vi "Get band variation.vi"(9 "# taps / position":i32=1, 10 "Bands 2":u16(ring)=2 items=["No Bands", "JC violin 200-7000 Flat (200-7000)", "JC violin (200-780-1740-2930-7000)", "JC violin (200-780-7000)", "MJ_Test (200-428-453-780-1740-2930-7000)"], 11 "Files":path[](array[path])=[path "/Users/crogers/Dropbox (Rogers)/Violin Stuff/PC ViolnData/SoundCard2/SoundCard2 ModalShop7/Raw/SoundCard2 ModalShop7 H_001_001.wfm", path "/Users/crogers/Dropbox (Rogers)/Violin Stuff/PC ViolnData/SoundCard2/SoundCard2 ModalShop7/Raw/SoundCard2 ModalShop7 H_001_002.wfm", path "/Users/crogers/Dropbox (Rogers)/Violin Stuff/PC ViolnData/SoundCard2/SoundCard2 ModalShop7/Raw/SoundCard2 ModalShop7 H_001_003.wfm", path "/Users/crogers/Dropbox (Rogers)/Violin Stuff/PC ViolnData/SoundCard2/SoundCard2 ModalShop7/Raw/SoundCard2 ModalShop7 H_001_004.wfm", path "/Users/crogers/Dropbox (Rogers)/Violin Stuff/PC ViolnData/SoundCard2/SoundCard2 ModalShop7/Raw/SoundCard2 ModalShop7 H_001_005.wfm", path "/Users/crogers/Dropbox (Rogers)/Violin Stuff/PC ViolnData/SoundCard2/SoundCard2 ModalShop7/Raw/SoundCard2 ModalShop7 H_001_006.wfm", path "/Users/crogers/Dropbox (Rogers)/Violin Stuff/PC ViolnData/SoundCard2/SoundCard2 ModalShop7/Raw/SoundCard2 ModalShop7 H_001_007.wfm", path "/Users/crogers/Dropbox (Rogers)/Violin Stuff/PC ViolnData/SoundCard2/SoundCard2 ModalShop7/Raw/SoundCard2 ModalShop7 H_001_008.wfm", path "/Users/crogers/Dropbox (Rogers)/Violin Stuff/PC ViolnData/SoundCard2/SoundCard2 ModalShop7/Raw/SoundCard2 ModalShop7 H_001_009.wfm", path "/Users/crogers/Dropbox (Rogers)/Violin Stuff/PC ViolnData/SoundCard2/SoundCard2 ModalShop7/Raw/SoundCard2 ModalShop7 H_001_010.wfm", path "/Users/crogers/Dropbox (Rogers)/Violin Stuff/PC ViolnData/SoundCard2/SoundCard2 ModalShop7/Raw/SoundCard2 ModalShop7 H_002_001.wfm", path "/Users/crogers/Dropbox (Rogers)/Violin Stuff/PC ViolnData/SoundCard2/SoundCard2 ModalShop7/Raw/SoundCard2 ModalShop7 H_002_002.wfm", path "/Users/crogers/Dropbox (Rogers)/Violin Stuff/PC ViolnData/SoundCard2/SoundCard2 ModalShop7/Raw/SoundCard2 ModalShop7 H_002_003.wfm", path "/Users/crogers/Dropbox (Rogers)/Violin Stuff/PC ViolnData/SoundCard2/SoundCard2 ModalShop7/Raw/SoundCard2 ModalShop7 H_002_004.wfm", path "/Users/crogers/Dropbox (Rogers)/Violin Stuff/PC ViolnData/SoundCard2/SoundCard2 ModalShop7/Raw/SoundCard2 ModalShop7 H_002_005.wfm", path "/Users/crogers/Dropbox (Rogers)/Violin Stuff/PC ViolnData/SoundCard2/SoundCard2 ModalShop7/Raw/SoundCard2 ModalShop7 H_002_006.wfm", path "/Users/crogers/Dropbox (Rogers)/Violin Stuff/PC ViolnData/SoundCard2/SoundCard2 ModalShop7/Raw/SoundCard2 ModalShop7 H_002_007.wfm", path "/Users/crogers/Dropbox (Rogers)/Violin Stuff/PC ViolnData/SoundCard2/SoundCard2 ModalShop7/Raw/SoundCard2 ModalShop7 H_002_008.wfm", path "/Users/crogers/Dropbox (Rogers)/Violin Stuff/PC ViolnData/SoundCard2/SoundCard2 ModalShop7/Raw/SoundCard2 ModalShop7 H_002_009.wfm", path "/Users/crogers/Dropbox (Rogers)/Violin Stuff/PC ViolnData/SoundCard2/SoundCard2 ModalShop7/Raw/SoundCard2 ModalShop7 H_002_010.wfm", path "/Users/crogers/Dropbox (Rogers)/Violin Stuff/PC ViolnData/SoundCard2/SoundCard2 ModalShop7/Raw/SoundCard2 ModalShop7 H_003_001.wfm", path "/Users/crogers/Dropbox (Rogers)/Violin Stuff/PC ViolnData/SoundCard2/SoundCard2 ModalShop7/Raw/SoundCard2 ModalShop7 H_003_002.wfm", path "/Users/crogers/Dropbox (Rogers)/Violin Stuff/PC ViolnData/SoundCard2/SoundCard2 ModalShop7/Raw/SoundCard2 ModalShop7 H_003_003.wfm", path "/Users/crogers/Dropbox (Rogers)/Violin Stuff/PC ViolnData/SoundCard2/SoundCard2 ModalShop7/Raw/SoundCard2 ModalShop7 H_003_004.wfm", path "/Users/crogers/Dropbox (Rogers)/Violin Stuff/PC ViolnData/SoundCard2/SoundCard2 ModalShop7/Raw/SoundCard2 ModalShop7 H_003_005.wfm", path "/Users/crogers/Dropbox (Rogers)/Violin Stuff/PC ViolnData/SoundCard2/SoundCard2 ModalShop7/Raw/SoundCard2 ModalShop7 H_003_006.wfm", path "/Users/crogers/Dropbox (Rogers)/Violin Stuff/PC ViolnData/SoundCard2/SoundCard2 ModalShop7/Raw/SoundCard2 ModalShop7 H_003_007.wfm", path "/Users/crogers/Dropbox (Rogers)/Violin Stuff/PC ViolnData/SoundCard2/SoundCard2 ModalShop7/Raw/SoundCard2 ModalShop7 H_003_008.wfm", path "/Users/crogers/Dropbox (Rogers)/Violin Stuff/PC ViolnData/SoundCard2/SoundCard2 ModalShop7/Raw/SoundCard2 ModalShop7 H_003_009.wfm", path "/Users/crogers/Dropbox (Rogers)/Violin Stuff/PC ViolnData/SoundCard2/SoundCard2 ModalShop7/Raw/SoundCard2 ModalShop7 H_003_010.wfm", path "/Users/crogers/Dropbox (Rogers)/Violin Stuff/PC ViolnData/SoundCard2/SoundCard2 ModalShop7/Raw/SoundCard2 ModalShop7 H_004_001.wfm", path "/Users/crogers/Dropbox (Rogers)/Violin Stuff/PC ViolnData/SoundCard2/SoundCard2 ModalShop7/Raw/SoundCard2 ModalShop7 H_004_002.wfm", path "/Users/crogers/Dropbox (Rogers)/Violin Stuff/PC ViolnData/SoundCard2/SoundCard2 ModalShop7/Raw/SoundCard2 ModalShop7 H_004_003.wfm", path "/Users/crogers/Dropbox (Rogers)/Violin Stuff/PC ViolnData/SoundCard2/SoundCard2 ModalShop7/Raw/SoundCard2 ModalShop7 H_004_004.wfm", path "/Users/crogers/Dropbox (Rogers)/Violin Stuff/PC ViolnData/SoundCard2/SoundCard2 ModalShop7/Raw/SoundCard2 ModalShop7 H_004_005.wfm", path "/Users/crogers/Dropbox (Rogers)/Violin Stuff/PC ViolnData/SoundCard2/SoundCard2 ModalShop7/Raw/SoundCard2 ModalShop7 H_004_006.wfm", path "/Users/crogers/Dropbox (Rogers)/Violin Stuff/PC ViolnData/SoundCard2/SoundCard2 ModalShop7/Raw/SoundCard2 ModalShop7 H_004_007.wfm", path "/Users/crogers/Dropbox (Rogers)/Violin Stuff/PC ViolnData/SoundCard2/SoundCard2 ModalShop7/Raw/SoundCard2 ModalShop7 H_004_008.wfm", path "/Users/crogers/Dropbox (Rogers)/Violin Stuff/PC ViolnData/SoundCard2/SoundCard2 ModalShop7/Raw/SoundCard2 ModalShop7 H_004_009.wfm", path "/Users/crogers/Dropbox (Rogers)/Violin Stuff/PC ViolnData/SoundCard2/SoundCard2 ModalShop7/Raw/SoundCard2 ModalShop7 H_004_010.wfm", path "/Users/crogers/Dropbox (Rogers)/Violin Stuff/PC ViolnData/SoundCard2/SoundCard2 ModalShop7/Raw/SoundCard2 ModalShop7 H_005_001.wfm", path "/Users/crogers/Dropbox (Rogers)/Violin Stuff/PC ViolnData/SoundCard2/SoundCard2 ModalShop7/Raw/SoundCard2 ModalShop7 H_005_002.wfm", path "/Users/crogers/Dropbox (Rogers)/Violin Stuff/PC ViolnData/SoundCard2/SoundCard2 ModalShop7/Raw/SoundCard2 ModalShop7 H_005_003.wfm", path "/Users/crogers/Dropbox (Rogers)/Violin Stuff/PC ViolnData/SoundCard2/SoundCard2 ModalShop7/Raw/SoundCard2 ModalShop7 H_005_004.wfm", path "/Users/crogers/Dropbox (Rogers)/Violin Stuff/PC ViolnData/SoundCard2/SoundCard2 ModalShop7/Raw/SoundCard2 ModalShop7 H_005_005.wfm", path "/Users/crogers/Dropbox (Rogers)/Violin Stuff/PC ViolnData/SoundCard2/SoundCard2 ModalShop7/Raw/SoundCard2 ModalShop7 H_005_006.wfm", path "/Users/crogers/Dropbox (Rogers)/Violin Stuff/PC ViolnData/SoundCard2/SoundCard2 ModalShop7/Raw/SoundCard2 ModalShop7 H_005_007.wfm", path "/Users/crogers/Dropbox (Rogers)/Violin Stuff/PC ViolnData/SoundCard2/SoundCard2 ModalShop7/Raw/SoundCard2 ModalShop7 H_005_008.wfm", path "/Users/crogers/Dropbox (Rogers)/Violin Stuff/PC ViolnData/SoundCard2/SoundCard2 ModalShop7/Raw/SoundCard2 ModalShop7 H_005_009.wfm", path "/Users/crogers/Dropbox (Rogers)/Violin Stuff/PC ViolnData/SoundCard2/SoundCard2 ModalShop7/Raw/SoundCard2 ModalShop7 H_005_010.wfm", path "/Users/crogers/Dropbox (Rogers)/Violin Stuff/PC ViolnData/SoundCard2/SoundCard2 ModalShop8/Raw/SoundCard2 ModalShop8 H_001_001.wfm", path "/Users/crogers/Dropbox (Rogers)/Violin Stuff/PC ViolnData/SoundCard2/SoundCard2 ModalShop8/Raw/SoundCard2 ModalShop8 H_001_002.wfm", path "/Users/crogers/Dropbox (Rogers)/Violin Stuff/PC ViolnData/SoundCard2/SoundCard2 ModalShop8/Raw/SoundCard2 ModalShop8 H_001_003.wfm", path "/Users/crogers/Dropbox (Rogers)/Violin Stuff/PC ViolnData/SoundCard2/SoundCard2 ModalShop8/Raw/SoundCard2 ModalShop8 H_001_004.wfm", path "/Users/crogers/Dropbox (Rogers)/Violin Stuff/PC ViolnData/SoundCard2/SoundCard2 ModalShop8/Raw/SoundCard2 ModalShop8 H_001_005.wfm", path "/Users/crogers/Dropbox (Rogers)/Violin Stuff/PC ViolnData/SoundCard2/SoundCard2 ModalShop8/Raw/SoundCard2 ModalShop8 H_001_006.wfm", path "/Users/crogers/Dropbox (Rogers)/Violin Stuff/PC ViolnData/SoundCard2/SoundCard2 ModalShop8/Raw/SoundCard2 ModalShop8 H_001_007.wfm", path "/Users/crogers/Dropbox (Rogers)/Violin Stuff/PC ViolnData/SoundCard2/SoundCard2 ModalShop8/Raw/SoundCard2 ModalShop8 H_001_008.wfm", path "/Users/crogers/Dropbox (Rogers)/Violin Stuff/PC ViolnData/SoundCard2/SoundCard2 ModalShop8/Raw/SoundCard2 ModalShop8 H_001_009.wfm", path "/Users/crogers/Dropbox (Rogers)/Violin Stuff/PC ViolnData/SoundCard2/SoundCard2 ModalShop8/Raw/SoundCard2 ModalShop8 H_001_010.wfm", path "/Users/crogers/Dropbox (Rogers)/Violin Stuff/PC ViolnData/SoundCard2/SoundCard2 ModalShop8/Raw/SoundCard2 ModalShop8 H_002_001.wfm", path "/Users/crogers/Dropbox (Rogers)/Violin Stuff/PC ViolnData/SoundCard2/SoundCard2 ModalShop8/Raw/SoundCard2 ModalShop8 H_002_002.wfm", path "/Users/crogers/Dropbox (Rogers)/Violin Stuff/PC ViolnData/SoundCard2/SoundCard2 ModalShop8/Raw/SoundCard2 ModalShop8 H_002_003.wfm", path "/Users/crogers/Dropbox (Rogers)/Violin Stuff/PC ViolnData/SoundCard2/SoundCard2 ModalShop8/Raw/SoundCard2 ModalShop8 H_002_004.wfm", path "/Users/crogers/Dropbox (Rogers)/Violin Stuff/PC ViolnData/SoundCard2/SoundCard2 ModalShop8/Raw/SoundCard2 ModalShop8 H_002_005.wfm", path "/Users/crogers/Dropbox (Rogers)/Violin Stuff/PC ViolnData/SoundCard2/SoundCard2 ModalShop8/Raw/SoundCard2 ModalShop8 H_002_006.wfm", path "/Users/crogers/Dropbox (Rogers)/Violin Stuff/PC ViolnData/SoundCard2/SoundCard2 ModalShop8/Raw/SoundCard2 ModalShop8 H_002_007.wfm", path "/Users/crogers/Dropbox (Rogers)/Violin Stuff/PC ViolnData/SoundCard2/SoundCard2 ModalShop8/Raw/SoundCard2 ModalShop8 H_002_008.wfm", path "/Users/crogers/Dropbox (Rogers)/Violin Stuff/PC ViolnData/SoundCard2/SoundCard2 ModalShop8/Raw/SoundCard2 ModalShop8 H_002_009.wfm", path "/Users/crogers/Dropbox (Rogers)/Violin Stuff/PC ViolnData/SoundCard2/SoundCard2 ModalShop8/Raw/SoundCard2 ModalShop8 H_002_010.wfm", path "/Users/crogers/Dropbox (Rogers)/Violin Stuff/PC ViolnData/SoundCard2/SoundCard2 ModalShop8/Raw/SoundCard2 ModalShop8 H_003_001.wfm", path "/Users/crogers/Dropbox (Rogers)/Violin Stuff/PC ViolnData/SoundCard2/SoundCard2 ModalShop8/Raw/SoundCard2 ModalShop8 H_003_002.wfm", path "/Users/crogers/Dropbox (Rogers)/Violin Stuff/PC ViolnData/SoundCard2/SoundCard2 ModalShop8/Raw/SoundCard2 ModalShop8 H_003_003.wfm", path "/Users/crogers/Dropbox (Rogers)/Violin Stuff/PC ViolnData/SoundCard2/SoundCard2 ModalShop8/Raw/SoundCard2 ModalShop8 H_003_004.wfm", path "/Users/crogers/Dropbox (Rogers)/Violin Stuff/PC ViolnData/SoundCard2/SoundCard2 ModalShop8/Raw/SoundCard2 ModalShop8 H_003_005.wfm", path "/Users/crogers/Dropbox (Rogers)/Violin Stuff/PC ViolnData/SoundCard2/SoundCard2 ModalShop8/Raw/SoundCard2 ModalShop8 H_003_006.wfm", path "/Users/crogers/Dropbox (Rogers)/Violin Stuff/PC ViolnData/SoundCard2/SoundCard2 ModalShop8/Raw/SoundCard2 ModalShop8 H_003_007.wfm", path "/Users/crogers/Dropbox (Rogers)/Violin Stuff/PC ViolnData/SoundCard2/SoundCard2 ModalShop8/Raw/SoundCard2 ModalShop8 H_003_008.wfm", path "/Users/crogers/Dropbox (Rogers)/Violin Stuff/PC ViolnData/SoundCard2/SoundCard2 ModalShop8/Raw/SoundCard2 ModalShop8 H_003_009.wfm", path "/Users/crogers/Dropbox (Rogers)/Violin Stuff/PC ViolnData/SoundCard2/SoundCard2 ModalShop8/Raw/SoundCard2 ModalShop8 H_003_010.wfm", path "/Users/crogers/Dropbox (Rogers)/Violin Stuff/PC ViolnData/SoundCard2/SoundCard2 ModalShop8/Raw/SoundCard2 ModalShop8 H_004_001.wfm", path "/Users/crogers/Dropbox (Rogers)/Violin Stuff/PC ViolnData/SoundCard2/SoundCard2 ModalShop8/Raw/SoundCard2 ModalShop8 H_004_002.wfm", path "/Users/crogers/Dropbox (Rogers)/Violin Stuff/PC ViolnData/SoundCard2/SoundCard2 ModalShop8/Raw/SoundCard2 ModalShop8 H_004_003.wfm", path "/Users/crogers/Dropbox (Rogers)/Violin Stuff/PC ViolnData/SoundCard2/SoundCard2 ModalShop8/Raw/SoundCard2 ModalShop8 H_004_004.wfm", path "/Users/crogers/Dropbox (Rogers)/Violin Stuff/PC ViolnData/SoundCard2/SoundCard2 ModalShop8/Raw/SoundCard2 ModalShop8 H_004_005.wfm", path "/Users/crogers/Dropbox (Rogers)/Violin Stuff/PC ViolnData/SoundCard2/SoundCard2 ModalShop8/Raw/SoundCard2 ModalShop8 H_004_006.wfm", path "/Users/crogers/Dropbox (Rogers)/Violin Stuff/PC ViolnData/SoundCard2/SoundCard2 ModalShop8/Raw/SoundCard2 ModalShop8 H_004_007.wfm", path "/Users/crogers/Dropbox (Rogers)/Violin Stuff/PC ViolnData/SoundCard2/SoundCard2 ModalShop8/Raw/SoundCard2 ModalShop8 H_004_008.wfm", path "/Users/crogers/Dropbox (Rogers)/Violin Stuff/PC ViolnData/SoundCard2/SoundCard2 ModalShop8/Raw/SoundCard2 ModalShop8 H_004_009.wfm", path "/Users/crogers/Dropbox (Rogers)/Violin Stuff/PC ViolnData/SoundCard2/SoundCard2 ModalShop8/Raw/SoundCard2 ModalShop8 H_004_010.wfm", path "/Users/crogers/Dropbox (Rogers)/Violin Stuff/PC ViolnData/SoundCard2/SoundCard2 ModalShop8/Raw/SoundCard2 ModalShop8 H_005_001.wfm", path "/Users/crogers/Dropbox (Rogers)/Violin Stuff/PC ViolnData/SoundCard2/SoundCard2 ModalShop8/Raw/SoundCard2 ModalShop8 H_005_002.wfm", path "/Users/crogers/Dropbox (Rogers)/Violin Stuff/PC ViolnData/SoundCard2/SoundCard2 ModalShop8/Raw/SoundCard2 ModalShop8 H_005_003.wfm", path "/Users/crogers/Dropbox (Rogers)/Violin Stuff/PC ViolnData/SoundCard2/SoundCard2 ModalShop8/Raw/SoundCard2 ModalShop8 H_005_004.wfm", path "/Users/crogers/Dropbox (Rogers)/Violin Stuff/PC ViolnData/SoundCard2/SoundCard2 ModalShop8/Raw/SoundCard2 ModalShop8 H_005_005.wfm", path "/Users/crogers/Dropbox (Rogers)/Violin Stuff/PC ViolnData/SoundCard2/SoundCard2 ModalShop8/Raw/SoundCard2 ModalShop8 H_005_006.wfm", path "/Users/crogers/Dropbox (Rogers)/Violin Stuff/PC ViolnData/SoundCard2/SoundCard2 ModalShop8/Raw/SoundCard2 ModalShop8 H_005_007.wfm", path "/Users/crogers/Dropbox (Rogers)/Violin Stuff/PC ViolnData/SoundCard2/SoundCard2 ModalShop8/Raw/SoundCard2 ModalShop8 H_005_008.wfm", path "/Users/crogers/Dropbox (Rogers)/Violin Stuff/PC ViolnData/SoundCard2/SoundCard2 ModalShop8/Raw/SoundCard2 ModalShop8 H_005_009.wfm", path "/Users/crogers/Dropbox (Rogers)/Violin Stuff/PC ViolnData/SoundCard2/SoundCard2 ModalShop8/Raw/SoundCard2 ModalShop8 H_005_010.wfm"]) -> (2 "sdev":dbl[](array[numeric]), 3 "mean":dbl[](array[numeric]))   [LabVIEW 2024]
uses:
  PreferencesControl.ctl
  <vilib>/Analysis/NI_AALBase.lvlib
panel:
  out "Histogram Graph":T1(graph)
  out "Bands 3":dbl[][](graph)
  out "Bands":cluster{dbl, "df":dbl, dbl[]}[](graph)
  out "Hammer Spectra":cluster{dbl, "df":dbl, "FFT {X}":dbl[]}[](graph)=[{0.0, "df"=1.0, "FFT {X}"=array[24001 elements]}]
  out "Microphone Spectra":cluster{"x0":dbl, "df":dbl, dbl[]}[](graph)=[{"x0"=0.0, "df"=1.0, array[24001 elements]}]
  out "Average FRF":cluster{dbl, "df":dbl, dbl[]}[](graph)=[{0.0, "df"=1.0, array[24001 elements]}, {0.0, "df"=1.0, array[24001 elements]}]
  out "Hammer":cluster{dbl, "dt":dbl, "Y":dbl[]}[](graph)=[{0.0, "dt"=2.0833333333333333e-05, "Y"=array[14400 elements]}]
  out "Microphone":cluster{dbl, "dt":dbl, "Y":dbl[]}[](graph)=[{0.0, "dt"=2.0833333333333333e-05, "Y"=array[14400 elements]}]
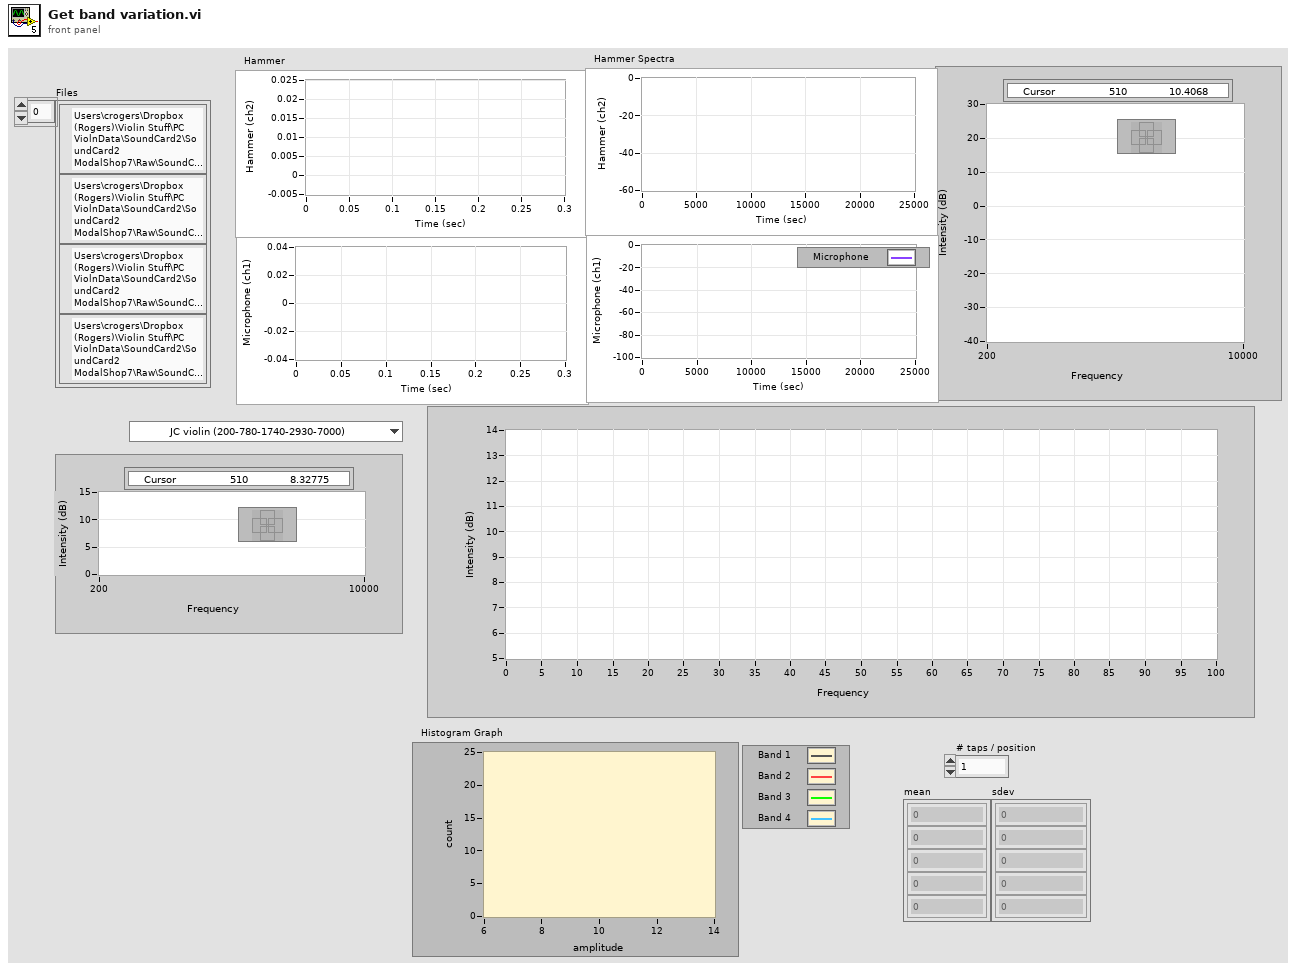
[diagram p1: front panel]
types:
  T1 = cluster{"X Values":dbl[], "Histogram: h(x)":i32[]}[]
  T2 = typedef "PreferencesControl.ctl" = cluster{"Name of test":string, "Date":timestamp, "Location":string, "Template":string, "Soundcard":string, "resolution":u16, "Sampling rate":u16, "Ch1 Gain ":dbl, "Ch2 Gain":dbl, "Sample time (s)":dbl, "Pre-trigger (s)":dbl, "Hammer Threshold":dbl, "Positions":i16, "Taps/Position":i16, "Set Names":string, "Freq resolution":dbl, "Hammer cutoff":dbl, "Mic cutoff":dbl, "Double bounce ":dbl, "Hammer Cal":dbl, "dB Offset":dbl, "Accel Cal":dbl, "Vibrometer Cal":dbl, "Mic Cal":dbl, "Output":u16, "Voltage Cal":dbl, "Vibrometer Port":refnum<visa-resource-name>, "Range":u16, "High Pass":u16, "Bandwidth":u16, "X Range":cluster{"Minimum":dbl, "Maximum":dbl, "Increment":dbl, "Minor Increment":dbl, "Start":dbl}[], "Y Range":cluster{"Minimum":dbl, "Maximum":dbl, "Increment":dbl, "Minor Increment":dbl, "Start":dbl}[], "dB Spread":dbl, "Trigger":u16, "Ch_1":u8, "Ch_2":u8, "flip?":bool, "60Hz":bool, "Time offset":dbl, "Piezo Cal":dbl, "Default Notes":string}
  T3 = cluster{"Name":string, "Color":u32, "Style":u8, "Point Style":u8, "Name Visible":bool, "Allow Drag":bool, "Cursor Mode":u32, "Plot":i32, "Index":i32, "Position":cluster{"X":dbl, "Y":dbl}, "X Scale":u32, "Y Scale":u32, "Watch Plots":i32[], "Watch All Plots":bool, "Plot Area":i32, "Label Offset":cluster{"X":dbl, "Y":dbl}}[]
  T4 = cluster{"Band ranges":dbl[][], "CoM":dbl[][], "Band Ave":dbl[][]}
  T5 = cluster{dbl, "df":dbl, "Power Spectrum (V^2 rms)":dbl[]}[]
  T6 = cluster{dbl, "df":dbl, "Power Spectrum (V^2 rms)":dbl[]}
  T7 = cluster{"X Values":dbl[], "Histogram: h(x)":i32[]}
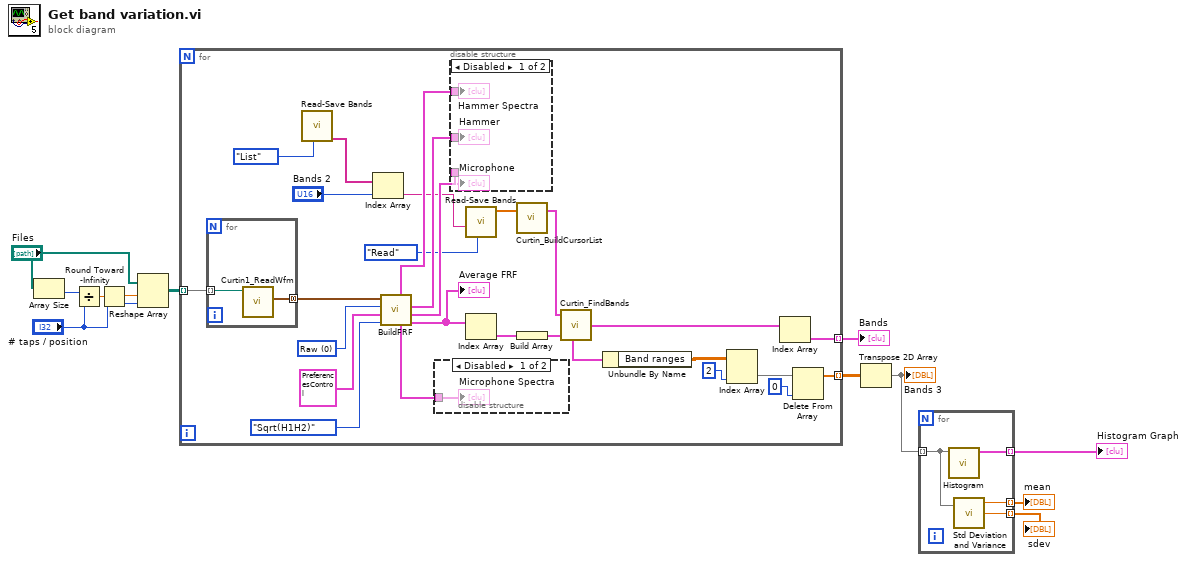
[diagram p0: block diagram]
diagram:
  n1 = Array Size(array="Files") -> (size(s)=w8:i32)
  n2 = Divide(x=w8, y="# taps / position") -> (x/y=w6:dbl)
  n3 = Round Toward -Infinity(1:w6) -> (0:w3:dbl)
  n4 = Reshape Array("Files", w3, "# taps / position") -> (w12:path[][])
  n5 = for {
    tunnel: w12 -> [w21] mode=indexing
    tunnel: [w19] -> w11 mode=indexing
    tunnel: [w14] -> w10 mode=indexing
    w38 = u16 0 items=["Raw", "Volts", "Units (Pa, N, mm/s etc)"] ("View")
    n6 = for {
      tunnel: [w45] -> w39 mode=concatenating
      tunnel: w21 -> [w44] mode=indexing
      n7 = call "Curtin1_ReadWfm.vi"("appended path"=w44) -> ("all waveforms in record"=w45:waveform(dbl)[])  [unwired: 9 in, 1 out]
    }
    n8 = call "Read-Save Bands.vi"("Task"=enum16{"Save", "Read", "List"}."List") -> ("file names"=w29:string[])  [unwired: 7 in, 3 out]
    n9 = Index Array(array=w29, index="Bands 2") -> (element=w28:string)
    n10 = call "BuildFRF.vi"("Method"=enum16{"Sqrt(H1H2)", "H1", "H2"}."Sqrt(H1H2)", "Settings"=T2 {"Name of test"="SoundCard2--SoundCard2 Focusrite", "Date"=timestamp(3723372723 s since 1904-01-01), "Location"="Home", "Template"="ScratchPad", "Soundcard"="Microphone (Scarlett 2i2 USB)", "resolution"=32, "Sampling rate"=48000, "Ch1 Gain "=0.0, "Ch2 Gain"=0.0, "Sample time (s)"=0.3, "Pre-trigger (s)"=0.001, "Hammer Threshold"=0.3327868852459017, "Positions"=1, "Taps/Position"=20, "Set Names"="H", "Freq resolution"=1.0, "Hammer cutoff"=0.0056410256410256415, "Mic cutoff"=0.25, "Double bounce "=0.01, "Hammer Cal"=1.0, "dB Offset"=0.0, "Accel Cal"=1.0, "Vibrometer Cal"=1.0, "Mic Cal"=1.0, "Output"=2, "Voltage Cal"=1.0, "Vibrometer Port"="ASRL27::INSTR", "Range"=20, "High Pass"=0, "Bandwidth"=25, "X Range"=[{"Minimum"=200.0, "Maximum"=10000.0, "Increment"=10.0, "Minor Increment"=100.0, "Start"=200.0}, {"Minimum"=0.0, "Maximum"=0.05, "Increment"=0.025, "Minor Increment"=0.0025, "Start"=0.0}, {"Minimum"=-0.02, "Maximum"=0.3, "Increment"=0.1, "Minor Increment"=0.01, "Start"=0.0}, {"Minimum"=150.0, "Maximum"=10000.0, "Increment"=10.0, "Minor Increment"=100.0, "Start"=1000.0}], "Y Range"=[{"Minimum"=-25.0, "Maximum"=0.0, "Increment"=5.0, "Minor Increment"=1.0, "Start"=-25.0}, {"Minimum"=-0.1, "Maximum"=1.0, "Increment"=0.25, "Minor Increment"=0.05, "Start"=0.0}, {"Minimum"=-1.0, "Maximum"=1.0, "Increment"=0.5, "Minor Increment"=0.1, "Start"=-1.0}, {"Minimum"=-12.0, "Maximum"=28.0, "Increment"=1.0, "Minor Increment"=0.25, "Start"=-12.0}], "dB Spread"=40.0, "Trigger"=0, "Ch_1"=1, "Ch_2"=2, "flip?"=FALSE, "60Hz"=FALSE, "Time offset"=0.0, "Piezo Cal"=1.0, "Default Notes"=""}, "View"=w38, "Data In"=w39) -> ("Average FRF"=w25:cluster{dbl, "df":dbl, dbl[]}[], "Microphone"=w33:cluster{dbl, "dt":dbl, "Y":dbl[]}[], "Hammer"=w34:cluster{dbl, "dt":dbl, "Y":dbl[]}[], "Microphone Spectra"=w32:cluster{"x0":dbl, "df":dbl, dbl[]}[], "Hammer Spectra"=w35:cluster{dbl, "df":dbl, "FFT {X}":dbl[]}[])  [unwired: 2 in, 1 out]
    "Average FRF" <- w25
    n11 = disable-structure shown="Disabled" {
      disable-tunnel: w32 -> [w40 _]
      frame Disabled {
        "Microphone Spectra" <- w40
      }
      frame Enabled {
      }
    }
    n12 = disable-structure shown="Disabled" {
      disable-tunnel: w35 -> [w43 _]
      disable-tunnel: w34 -> [w42 _]
      disable-tunnel: w33 -> [w41 _]
      frame Disabled {
        "Microphone" <- w41
        "Hammer" <- w42
        "Hammer Spectra" <- w43
      }
      frame Enabled {
      }
    }
    n13 = call "Read-Save Bands.vi"("Task"=enum16{"Save", "Read", "List"}."Read", "Name"=w28) -> ("Frequencies"=w24:dbl[])  [unwired: 6 in, 3 out]
    n14 = Index Array(array=w25) -> (element=w23:cluster{dbl, "df":dbl, dbl[]})  [unwired: 1 in]
    n15 = call "Curtin_BuildCursorList.vi"("Fctr"=w24) -> ("Cursor List"=w27:T3)  [unwired: 1 in, 1 out]
    n16 = Build Array(w23) -> (w22:cluster{dbl, "df":dbl, dbl[]}[])
    n17 = call "Curtin_FindBands.vi"("CrsrList"=w27, "Magnitude"=w22) -> ("Raw Data"=w18:T4, "Filter"=w20:T5)  [unwired: 2 in, 2 out]
    n18 = Unbundle By Name(w18) -> ("Band ranges"=w17:dbl[][])
    n19 = Index Array(array=w17, index (col)=2 ("disabled index (col)")) -> (element=w16:dbl[])  [unwired: 1 in]
    n20 = Index Array(array=w20) -> (element=w19:T6)  [unwired: 1 in]
    n21 = Delete From Array(array=w16, index=0 ("length")) -> (array with subset deleted=w14:dbl[])  [unwired: 1 in, 1 out]
  }
  "Bands" <- w11
  n22 = Transpose 2D Array(2D array=w10) -> (transposed array=w5:dbl[][])
  "Bands 3" <- w5
  n23 = for {
    tunnel: w5 -> [w48] mode=indexing
    tunnel: [w49] -> w4 mode=indexing
    tunnel: [w47] -> w2 mode=indexing
    tunnel: [w46] -> w1 mode=indexing
    n24 = call <vilib>:"Histogram.vi"("X"=w48) -> ("Histogram Graph"=w49:T7)  [unwired: 7 in, 3 out]
    n25 = call <vilib>:"Std Deviation and Variance.vi"("X"=w48) -> ("mean"=w47:dbl, "standard deviation"=w46:dbl)  [unwired: 1 in, 1 out]
  }
  "Histogram Graph" <- w4
  "mean" <- w2
  "sdev" <- w1
